vi "Чтениемассива.vi"() -> ()   [LabVIEW 2017]
panel:
  out "array":dbl[][](array[numeric])
  out "text":string
  in  "file (use dialog)":path
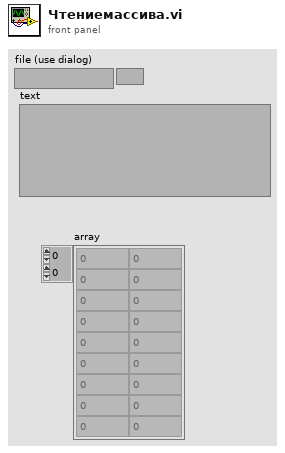
[diagram p1: front panel]
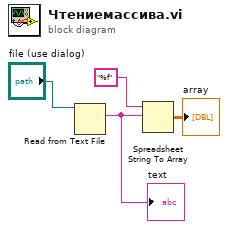
[diagram p0: block diagram]
diagram:
  n1 = Read from Text File(file (use dialog)="file (use dialog)") -> (text=w3:string)  [unwired: 3 in, 3 out]
  "text" <- w3
  n2 = Spreadsheet String To Array(format string="%f", spreadsheet string=w3) -> (array=→"array":dbl[][])  [unwired: 2 in]
